vi "Sensor Read.vi"(8 "Error In":errorcluster, 9 "Pressure Freq":dbl=30.0, 10 "Temperature Freq":dbl=30.0, 11 "Sampling Time":dbl=1.0) -> (0 "Error Out":errorcluster, 1 "Temperature Data":waveform(dbl)[](array[waveform]), 2 "Photodiode Data":waveform(dbl)[](array[waveform]), 3 "Pressure Data":waveform(dbl)[](array[waveform]))   [LabVIEW 2016]
uses:
  <vilib>/DAQmx/read.llb/DAQmx Read (Analog 1D Wfm NChan NSamp).vi
  <vilib>/DAQmx/read.llb/DAQmx Read (Analog 1D Wfm NChan 1Samp).vi
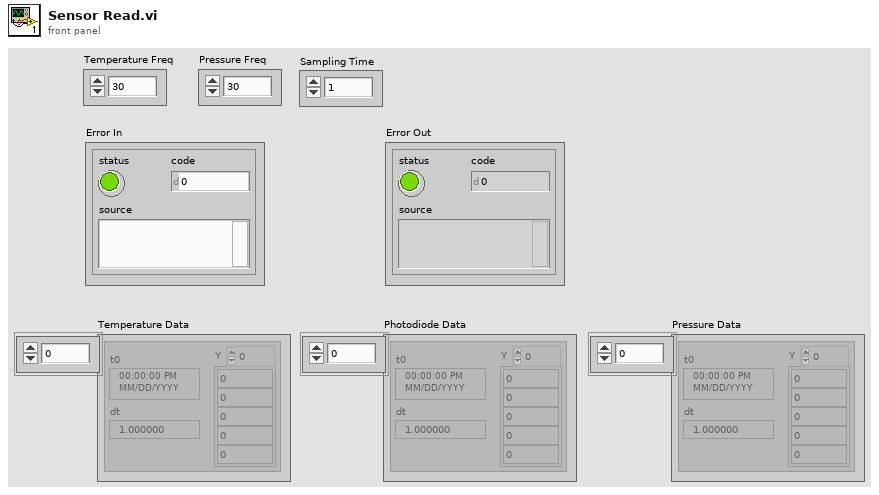
[diagram p1: front panel]
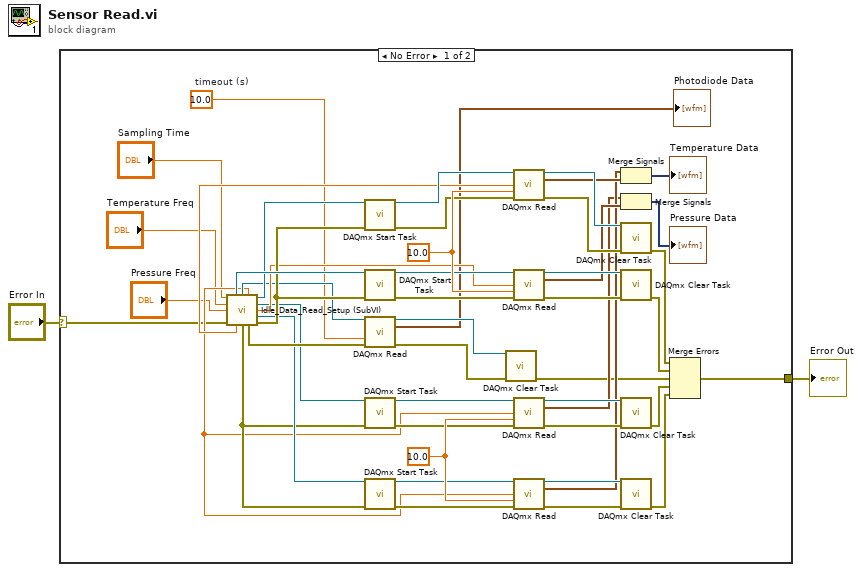
[diagram p0: block diagram]
diagram:
  n1 = case shown="No Error" "Error In" {
    selector: "Error In" -> [w6 w52]
    tunnel: [w31 w52] -> w2
    frame No Error {
      w24 = 10.0 ("timeout")
      w26 = 10.0  # timeout (s)
      w49 = 10.0 ("timeout")
      n2 = call "Idle_Data_Read_Setup (SubVI).vi"("Sampling Time"="Sampling Time", "Temperature Freq"="Temperature Freq", "Pressure Freq"="Pressure Freq", "error in (no error)"=w6) -> ("Pressure Task 2"=w48:refnum<k21>, "task out"=w29:refnum<k21>, "Samples Per Channel"=w13:dbl, "Refnum out"=w47:refnum<k21>, "Pressure Task"=w12:refnum<k21>, "Pressure Samples"=w35:dbl, "Temperature Task"=w23:refnum<k21>, "Temperature Samples"=w34:dbl, 13:"error out"=w14:errorcluster, "error out 2"=w30:errorcluster, 15:"error out"=w36:errorcluster)  [unwired: 1 in]
      n3 = call <vilib>:"DAQmx Start Task.vi"("task/channels in"=w47, "error in"=w36) -> ("task out"=w43:refnum<k21>, "error out"=w44:errorcluster)  [unwired: 12 out]
      n4 = call <vilib>:"DAQmx Start Task.vi"("task/channels in"=w48, "error in"=w36) -> ("task out"=w39:refnum<k21>, "error out"=w40:errorcluster)  [unwired: 12 out]
      n5 = call-poly <vilib>:"DAQmx Read.vi"("task/channels in"=w29, "timeout"=w26, "error in"=w30) -> ("task out"=w28:refnum<k21>, "data"=→"Photodiode Data":waveform(dbl)[], "error out"=w27:errorcluster)  [unwired: 10 in]
      n6 = call <vilib>:"DAQmx Start Task.vi"("task/channels in"=w12, "error in"=w14) -> ("task out"=w15:refnum<k21>, "error out"=w16:errorcluster)  [unwired: 12 out]
      n7 = call <vilib>:"DAQmx Start Task.vi"("task/channels in"=w23, "error in"=w14) -> ("task out"=w19:refnum<k21>, "error out"=w20:errorcluster)  [unwired: 12 out]
      n8 = call <vilib>:"DAQmx Clear Task.vi"("task in"=w28, "error in"=w27) -> ("error out"=w5:errorcluster)  [unwired: 13 in]
      n9 = call-poly <vilib>:"DAQmx Read.vi"("task/channels in"=w43, "number of samples per channel"=w34, "timeout"=w49, "error in"=w44) -> ("task out"=w46:refnum<k21>, "data"=w33:waveform(dbl)[], "error out"=w45:errorcluster)  [unwired: 9 out]
      n10 = call-poly <vilib>:"DAQmx Read.vi"("task/channels in"=w39, "number of samples per channel"=w35, "timeout"=w49, "error in"=w40) -> ("task out"=w42:refnum<k21>, "data"=w32:waveform(dbl)[], "error out"=w41:errorcluster)  [unwired: 9 out]
      n11 = call-poly <vilib>:"DAQmx Read.vi"("task/channels in"=w15, "number of samples per channel"=w13, "timeout"=w24, "error in"=w16) -> ("task out"=w18:refnum<k21>, "data"=w7:waveform(dbl)[], "error out"=w17:errorcluster)  [unwired: 9 out]
      n12 = call-poly <vilib>:"DAQmx Read.vi"("task/channels in"=w19, "number of samples per channel"=w13, "timeout"=w24, "error in"=w20) -> ("task out"=w22:refnum<k21>, "data"=w8:waveform(dbl)[], "error out"=w21:errorcluster)  [unwired: 9 out]
      n13 = Merge Signals(w8, w33) -> (→"Temperature Data":dynamicdata)
      n14 = Merge Signals(w7, w32) -> (→"Pressure Data":dynamicdata)
      n15 = call <vilib>:"DAQmx Clear Task.vi"("task in"=w46, "error in"=w45) -> ("error out"=w37:errorcluster)  [unwired: 13 out]
      n16 = call <vilib>:"DAQmx Clear Task.vi"("task in"=w42, "error in"=w41) -> ("error out"=w38:errorcluster)  [unwired: 13 out]
      n17 = call <vilib>:"DAQmx Clear Task.vi"("task in"=w18, "error in"=w17) -> ("error out"=w4:errorcluster)  [unwired: 13 out]
      n18 = call <vilib>:"DAQmx Clear Task.vi"("task in"=w22, "error in"=w21) -> ("error out"=w3:errorcluster)  [unwired: 13 out]
      n19 = Merge Errors(w37, w38, w5, w4, w3) -> (w31:errorcluster)
    }
    frame Error {
    }
  }
  "Error Out" <- w2
